vi "GetControlRefs.vi"(11 "clControlRefs In":T1) -> (3 "clControlRefs Out":T1)   [LabVIEW 2014, in "Framework.lvlib"]
uses:
  Framework.lvlib
  TypeDefs/clFrontPanelControlRefs.ctl
  TypeDefs/clEventConfig.ctl
  Modules/PmuImpairPlugins/PmuImpairPluginBase_class/TypeDefs/clImpairConfig.ctl
  Modules/PmuImpairPlugins/PmuImpairPluginBase_class/PmuImpairPluginBase.lvclass
panel:
  # "When you add a control \non the front panel, add a\nreference for it in this\ntype def.  This cluster\nwill hold all of the refer-\nences to the front panel\ncontrols in order to pass\nthese control references \nto subvis."
  # "When you add a control \non the front panel, add a\nreference for it in this\ntype def.  This cluster\nwill hold all of the refer-\nences to the front panel\ncontrols in order to pass\nthese control references \nto subvis."
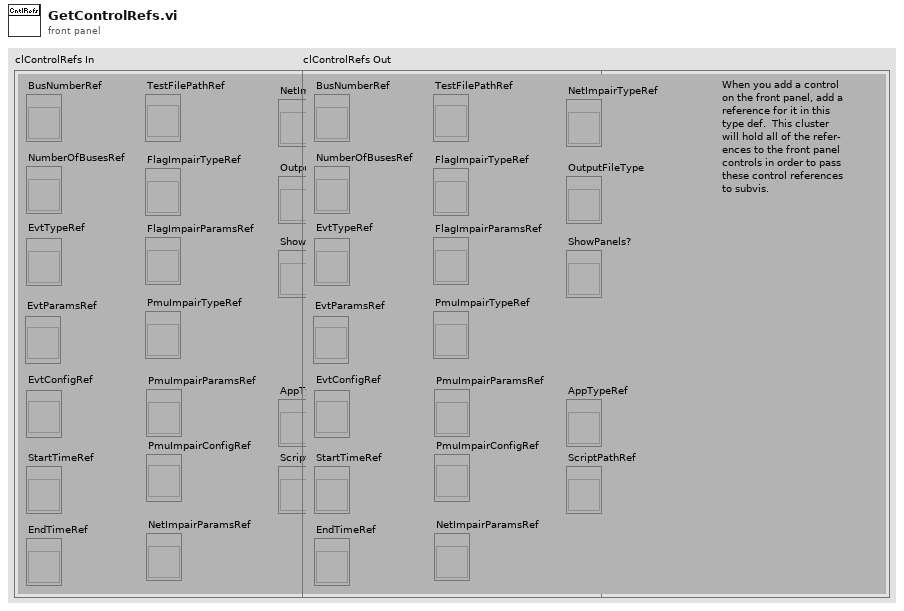
[diagram p1: front panel]
types:
  T1 = typedef "Framework.lvlib/clFrontPanelControlRefs.ctl" = cluster{"TestFilePathRef":refnum<vi>, "BusNumberRef":refnum<vi>, "NumberOfBusesRef":refnum<vi>, "EvtTypeRef":refnum<vi>, "EvtParamsRef":refnum<vi>, "EvtConfigRef":refnum<vi>, "StartTimeRef":refnum<vi>, "EndTimeRef":refnum<vi>, "PmuImpairTypeRef":refnum<vi>, "PmuImpairParamsRef":refnum<vi>, "NetImpairParamsRef":refnum<vi>, "FlagImpairTypeRef":refnum<vi>, "FlagImpairParamsRef":refnum<vi>, "NetImpairTypeRef":refnum<vi>, "OutputFileType":refnum<vi>, "PmuImpairConfigRef":refnum<vi>, "AppTypeRef":refnum<vi>, "ScriptPathRef":refnum<vi>, "ShowPanels?":refnum<vi>}
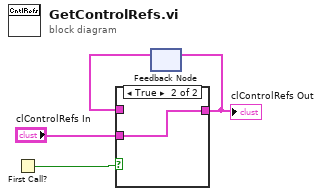
[diagram p0: block diagram]
diagram:
  n1 = First Call?() -> (First Call?: T/F=w4:bool)
  n2 = feedback #1() -> (w1:T1)  [unwired: 1 in]
  n3 = case shown="True" w4 {
    tunnel: "clControlRefs In" -> [_ w6]
    tunnel: [w5 w6] -> w2
    tunnel: w1 -> [w5 _]
    frame False {
    }
    frame True {
    }
  }
  "clControlRefs Out" <- w2
  n4 = feedback-in #1(w2) -> ()
